vi "ErrorHandling.Fglb.Add.vi"(7 "Event source":T1, 8 "error in (no error)":errorcluster, 10 "Error in":T2) -> (0 "error out":errorcluster, 1 "changed?":bool)   [LabVIEW 2016]
uses:
  CitTemplate/citTemplate.errData.ctl
  EventLog/EventLog.EventSource.ctl
  ErrorHandling.Fglb.Action.ctl
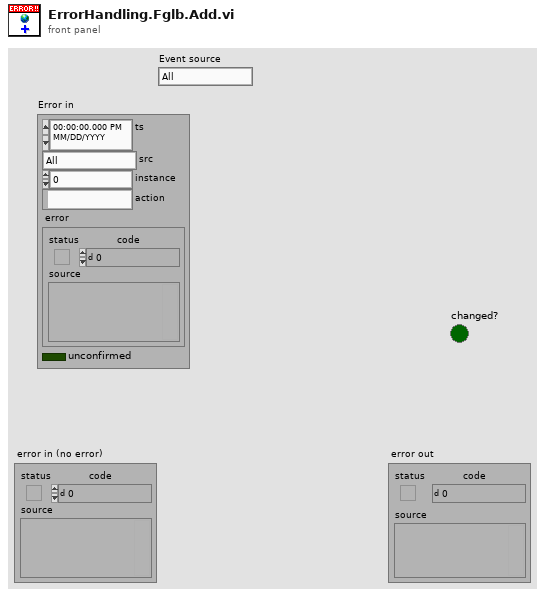
[diagram p1: front panel]
types:
  T1 = typedef "EventLog.EventSource.ctl" = enum16{"All", "Gui", "Ref", "File", "Arch", "Seq", "CPX", "DB", "Laser", "Scan.P", "Scan.O", "PLC"}
  T2 = typedef "citTemplate.errData.ctl" = cluster{"ts":timestamp, "src":T1, "instance":i32, "action":string, "error":errorcluster, "unconfirmed":bool}
  T3 = typedef "ErrorHandling.Fglb.Action.ctl" = enum16{"init", "add", "clear", "confirm", "check", "get"}
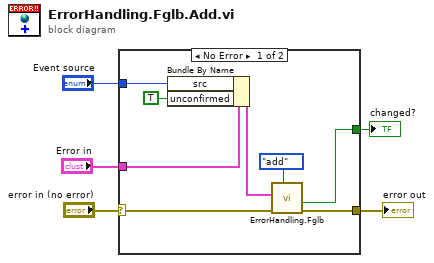
[diagram p0: block diagram]
diagram:
  n1 = case shown="No Error" "error in (no error)" {
    selector: "error in (no error)" -> [w11 w14]
    tunnel: [w12 w14] -> w5
    tunnel: "Error in" -> [w9 _]
    tunnel: "Event source" -> [w7 _]
    tunnel: [w10 _] -> w1
    frame No Error {
      n2 = Bundle By Name(cluster=w9, "src"=w7, "unconfirmed"=TRUE) -> (w8:T2)
      n3 = call "ErrorHandling.Fglb.vi"("Action"=ErrorHandling.Fglb.Action."add", "error in (no error)"=w11, "Error in"=w8) -> ("error out"=w12:errorcluster, "changed"=w10:bool)  [unwired: 6 in, 1 out]
    }
    frame Error {
    }
  }
  "error out" <- w5
  "changed?" <- w1
